vi "imaq_alloc.vi"() -> ()   [LabVIEW 2025]
uses:
  <vilib>/vision/NI_Vision_Development_Module.lvlib
panel:
  in  "Stop":bool
  out "Second Fill":dbl
  out "First Fill":dbl
  in  "Continue":bool
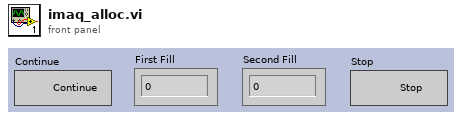
[diagram p1: front panel]
types:
  T1 = typedef "IMAQ Image.ctl" = refnum<image>
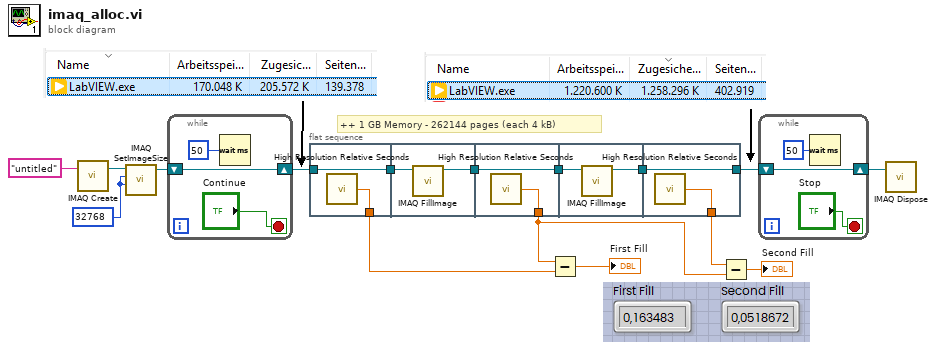
[diagram p0: block diagram]
diagram:
  w14 = 32768 ("X Resolution")
  # "++ 1 GB Memory - 262144 pages (each 4 kB)"
  n1 = call "IMAQ Create"("Image Name"="untitled") -> ("New Image"=w15:T1)  [unwired: 4 in, 1 out]
  n2 = call "IMAQ SetImageSize"("Y Resolution"=w14, "X Resolution"=w14, "Image"=w15) -> ("Image Out"=w13:T1)  [unwired: 2 in, 1 out]
  n3 = while {
    shift-right: [w17] -> w6
    shift-left: w13 -> [w17]
    stop <- "Continue" stop-if-true
    n4 = Wait (ms)(milliseconds to wait=u32 50) -> ()  [unwired: 1 out]
  }
  n5 = flat-sequence {
    tunnel: [w21] -> w12
    tunnel: [w20] -> w7
    tunnel: w6 -> [w20]
    tunnel: w7 -> [w23]
    tunnel: [w22] -> w4
    tunnel: [w25] -> w10
    tunnel: [w24] -> w5
    tunnel: w4 -> [w24]
    tunnel: w5 -> [w27]
    tunnel: [w26] -> w3
    tunnel: [w29] -> w11
    tunnel: [w28] -> w2
    tunnel: w3 -> [w28]
    frame #0 {
      n6 = call <vilib>:"High Resolution Relative Seconds.vi"() -> ("relative seconds"=w21:dbl)
    }
    frame #1 {
      n7 = call "IMAQ FillImage"("Image"=w23) -> ("Image Out"=w22:T1)  [unwired: 9 in, 1 out]
    }
    frame #2 {
      n8 = call <vilib>:"High Resolution Relative Seconds.vi"() -> ("relative seconds"=w25:dbl)
    }
    frame #3 {
      n9 = call "IMAQ FillImage"("Image"=w27) -> ("Image Out"=w26:T1)  [unwired: 9 in, 1 out]
    }
    frame #4 {
      n10 = call <vilib>:"High Resolution Relative Seconds.vi"() -> ("relative seconds"=w29:dbl)
    }
  }
  n11 = Subtract(x=w10, y=w12) -> (x-y=→"First Fill":dbl)
  n12 = Subtract(x=w11, y=w10) -> (x-y=→"Second Fill":dbl)
  n13 = while {
    shift-right: [w30] -> w1
    shift-left: w2 -> [w30]
    stop <- "Stop" stop-if-true
    n14 = Wait (ms)(milliseconds to wait=u32 50) -> ()  [unwired: 1 out]
  }
  n15 = call "IMAQ Dispose"("Image"=w1) -> ()  [unwired: 5 in, 1 out]
